vi "SingleCounterGated.vi"(7 "Acquisition time [s]":dbl=0.1 format="%.3f", 8 "error in":errorcluster, 9 "Gate input":tag="/Dev1/PFI24" caption="External Timing Source", 10 "Gate":tag="Dev1/ctr3", 11 "Counter":tag="Dev1/ctr0") -> (0 "error out":errorcluster, 2 "counts/s":dbl=10.0, 3 "counts":u32=1)   [LabVIEW 2014]
doc: "I. Description:\nThis example demonstrates how to count digital events on a Counter Input Channel. The Initial Count, Count Direction, and Edge are all configurable. This example also shows how to use a secondary counter and a digital input line to count events for a specified amount of time, following an external digital trigger.\n\nEdges are counted on the primary counter's default input terminal (refer to section IV, I/O Connections Overview, for more information), but it could easily be modified to count edges on a PFI or RTSI line. \n\nII. Instructions for Running:\n1. Select the Physical Channel that corresponds to the counter you want to count edges on the DAQ device. (This counter is called the Input Counter.)\n2. Enter the Initial Count, Count Direction, and measurement Edge to specify how you want the counter to count. Additionally, you can change the input terminal where events are counted using the channel property node.\n3. Select the Physical Channel that corresponds to the secondary counter you want to generate a single pulse on the DAQ device. (This counter is called the Gating Counter.)\n4. Enter the Gate Length, Idle State, and Initial Delay to specify how you want the gate signal to be generated.\n5. Select the source for the Digital Start Trigger and the on which to trigger.\n\nIII. Block Diagram Steps:\n1. Create a Counter Input channel to Count Events. The Edge parameter is used to determine if the counter will increment on rising or falling edges.\n2. Create a Counter Output channel to produce a Pulse in terms of Time. If the Idle State of the pulse is set to low, the state of the line will begin low and remain low after the generation is stopped.\n3. Call the DAQmx Start Trigger VI to configure the pulse to begin on a digital trigger.\n4. Call the Start VI in each task to arm the counters and begin counting or generating. The input counter will be preloaded with the Initial Count. The pulse will not begin until the generating counter receives a digital trigger and after the Initial Delay (in seconds) has expired.\n5. Use the Wait Until Done VI to ensure the entire gate pulse is generated before ending the task.\n6. Call the DAQmx Read VI to poll the input counter after the gate pulse generation has finished.\n7. Call the Clear Task VI to clear each Task.\n8. Use the popup dialog box to display an error, if any.\n\nIV. I/O Connections Overview:\nThe input counter will count edges on the input terminal of the counter specified in the left Physical Channel I/O control. The gating counter will generate a digital pulse on the output terminal of the counter specified in the right Physical Channel I/O control. Connect the default output line of the gating counter to the default gate line of the input counter. This will allow the gating counter to control when the input counter can count events.\n\nIn this example the input counter will count edges on the default input terminal on ctr0, and the gating counter will generate a digital pulse on the default output terminal on ctr1. Connect your start trigger source to the appropriate connection specified by \"Start Trigger Source\" on the front panel. \n\nFor more information on the default counter input and output terminals for your device, open the NI-DAQmx Help, and refer to Counter Signal Connections found under the Device Considerations book in the table of contents."
uses:
  <vilib>/DAQmx/read.llb/DAQmx Read (Counter U32 1Chan 1Samp).vi
  <vilib>/DAQmx/create/channels.llb/DAQmx Create Channel (CI-Count Edges).vi
  <vilib>/DAQmx/create/channels.llb/DAQmx Create Channel (CO-Pulse Generation-Time).vi
  <vilib>/DAQmx/configure/timing.llb/DAQmx Timing (Implicit).vi
  <vilib>/DAQmx/miscellaneous.llb/DAQmx Fill In Error Info.vi
  <resource>/objmgr/daqmx.rc
panel:
  # "ctr0"
  # "PFI15 (correct PFI address is given in manual;\nas long as this address is used, no hard wiring is required)"
  # "ctr3"
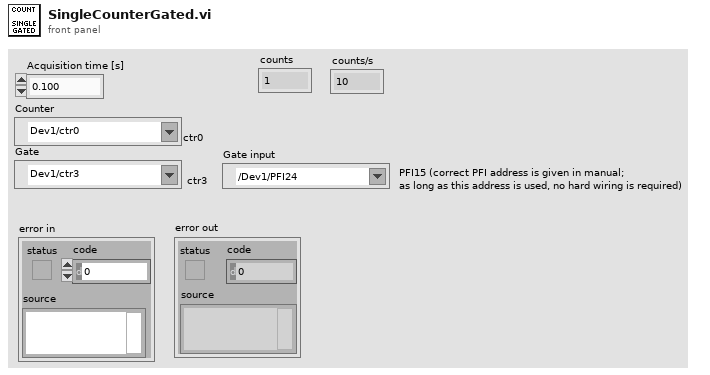
[diagram p1: front panel]
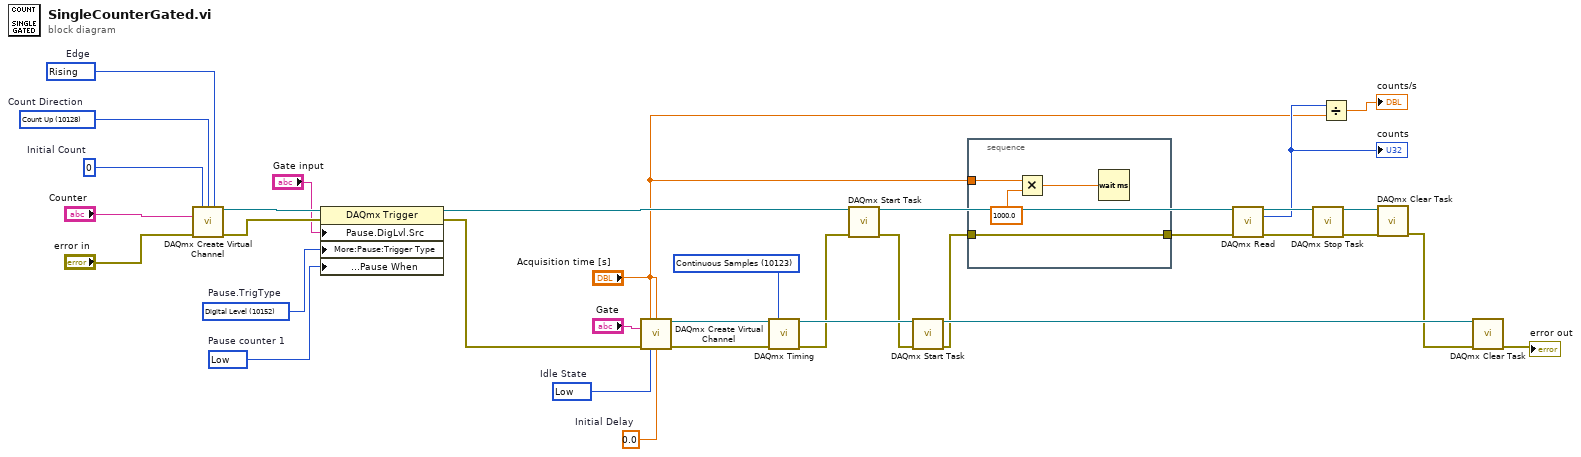
[diagram p0: block diagram]
diagram:
  w24 = 10214 items=["High"=10192, "Low"=10214]  # Pause counter 1
  w26 = 10123 items=["Finite Samples"=10178, "Continuous Samples"=10123, "Hardware Timed Single Point"=12522] ("sample mode")
  w30 = 0.0  # Initial Delay
  w31 = 10214 items=["High"=10192, "Low"=10214]  # Idle State
  w32 = u32 0  # Initial Count
  w33 = 10128 items=["Count Up"=10128, "Count Down"=10124, "Externally Controlled"=10326]  # Count Direction
  w34 = 10280 items=["Rising"=10280, "Falling"=10171]  # Edge
  w3 = 10152 items=["Analog Level"=10101, "Analog Window"=10103, "Digital Level"=10152, "Digital Pattern"=10398, "None"=10230]  # Pause.TrigType
  n1 = call-poly <vilib>:"DAQmx Create Virtual Channel.vi"("initial count"=w32, "count direction"=w33, "edge"=w34, "counter"="Counter", "error in"="error in") -> ("task out"=w22:refnum<k21>, "error out"=w23:errorcluster)  [unwired: 9 in]
  n2 = property class="DAQmx Trigger"(reference=w22, error in=w23, "Pause.DigLvl.Src"="Gate input", "More:Pause:Trigger Type"=w3, "More:Pause:Digital Level:Pause When"=w24) -> (reference out=w25:refnum<k21>, error out=w15:errorcluster)
  n3 = call-poly <vilib>:"DAQmx Create Virtual Channel.vi"("high time"="Acquisition time [s]", "low time"="Acquisition time [s]", "counter"="Gate", "error in"=w15, "idle state"=w31, "initial delay"=w30) -> ("task out"=w27:refnum<k21>, "error out"=w29:errorcluster)  [unwired: 8 in]
  n4 = call-poly <vilib>:"DAQmx Timing.vi"("task/channels in"=w27, "sample mode"=w26, "error in"=w29) -> ("task out"=w28:refnum<k21>, "error out"=w11:errorcluster)  [unwired: 11 in]
  n5 = call <vilib>:"DAQmx Start Task.vi"("task/channels in"=w25, "error in"=w11) -> ("task out"=w19:refnum<k21>, "error out"=w10:errorcluster)  [unwired: 12 in]
  n6 = call <vilib>:"DAQmx Start Task.vi"("task/channels in"=w28, "error in"=w10) -> ("task out"=w21:refnum<k21>, "error out"=w9:errorcluster)  [unwired: 12 in]
  n7 = stacked-sequence {
    tunnel: [w38] -> w18
    tunnel: w9 -> [w38]
    tunnel: "Acquisition time [s]" -> [w35]
    frame #0 {
      n8 = Multiply(x=w35, y=1000.0) -> (x*y=w37:dbl)
      n9 = Wait (ms)(milliseconds to wait=w37) -> ()  [unwired: 1 out]
    }
  }
  n10 = call-poly <vilib>:"DAQmx Read.vi"("task/channels in"=w19, "error in"=w18) -> ("task out"=w17:refnum<k21>, "data"=w16:u32, "error out"=w14:errorcluster)  [unwired: 11 in]
  "counts" <- w16
  n11 = call <vilib>:"DAQmx Stop Task.vi"("task/channels in"=w17, "error in"=w14) -> ("task out"=w20:refnum<k21>, "error out"=w13:errorcluster)  [unwired: 12 in]
  n12 = Divide(x=w16, y="Acquisition time [s]") -> (x/y=→"counts/s":dbl)
  n13 = call <vilib>:"DAQmx Clear Task.vi"("task in"=w20, "error in"=w13) -> ("error out"=w12:errorcluster)  [unwired: 13 in]
  n14 = call <vilib>:"DAQmx Clear Task.vi"("task in"=w21, "error in"=w12) -> ("error out"=→"error out":errorcluster)  [unwired: 13 in]
